vi "Append Attributes.vi"(9 "attributes":variant, 10 "Indent":string, 11 "String in":string) -> (2 "Indent dup":string, 3 "String out":string)   [LabVIEW 2013, in "Caraya.lvlib" / "Test Report.Event.lvclass"]
uses:
  Test Report.Event.lvclass
  MsgSerializer/MsgSerializer.lvclass
  Test Report/Test Report.lvclass
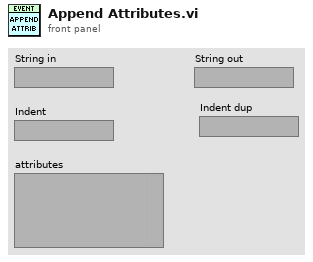
[diagram p1: front panel]
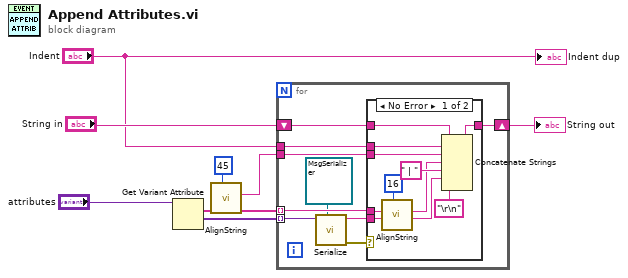
[diagram p0: block diagram]
diagram:
  n1 = Get Variant Attribute(Variant="attributes") -> (names=w3:string[], values=w4:variant[])  [unwired: 3 in, 2 out]
  n2 = call "AlignString.vi"("min length"=45 ("y")) -> ("Output"=w7:string)  [unwired: 10 in]
  n3 = for {
    shift-right: [w17] -> w5
    shift-left: "String in" -> [w16]
    tunnel: w3 -> [w13] mode=indexing
    tunnel: w4 -> [w12] mode=indexing
    tunnel: "Indent" -> [w15]
    tunnel: w7 -> [w14]
    n4 = call-dynamic "Serialize.vi"("MsgSerializer"=refnum<class "MsgSerializer.lvclass"> refnum ("Caraya.lvlib:MsgSerializer.lvclass"), "Value"=w12) -> ("error out"=w10:errorcluster, "Serialized Message"=w11:string)  [unwired: 8 in]
    n5 = case shown="No Error" w10 {
      tunnel: [w26 w28] -> w17
      tunnel: w16 -> [w27 w28]
      tunnel: w15 -> [w25 _]
      tunnel: w14 -> [w24 _]
      tunnel: w13 -> [w20 _]
      tunnel: w11 -> [w23 _]
      frame No Error {
        n6 = call "AlignString.vi"("min length"=16, "Input"=w20) -> ("Output"=w19:string)  [unwired: 9 in]
        n7 = Concatenate Strings(w27, w25, w24, w19, " | " ("string"), w23, "\r\n" ("format string")) -> (w26:string)
      }
      frame Error {
      }
    }
  }
  "String out" <- w5
  "Indent dup" <- "Indent"
